vi "attribute_write_boolean.vi"(5 "Repeated Capability":string, 7 "Attribute":T1={"Identifier"="", "Descriptive name"="", "Data Type"=enum."Integer 32", "Command"="", "Access"=2, "Range Table"="", "Read Callback"="", "Write Callback"="", "Range Callback"="", "Check Callback"="", "Rngtable Callback"="", "Coerce Callback"="", "Supported Models"="", "Instrument Options"="", "Repeated Capabilities"="", "Check Status Callback"="", "Index"=0, "Flag: OPC Wait"=FALSE, "Flag: Dont check status"=FALSE, "Flag: Cache Only"=FALSE} {"Access" items=["Read Only", "Write Only", "Read/Write"]}, 8 "error in":errorcluster, 10 "boolean in":bool, 11 "VISA resource name":refnum<visa-resource-name>) -> (0 "error out":errorcluster, 3 "VISA resource name out":refnum<visa-resource-name>)   [LabVIEW 2014, in "rszvl_rsidr_core.lvlib"]
uses:
  rszvl_rsidr_core.lvlib
  type_Attribute.ctl
  type_Attribute_Data_Type.ctl
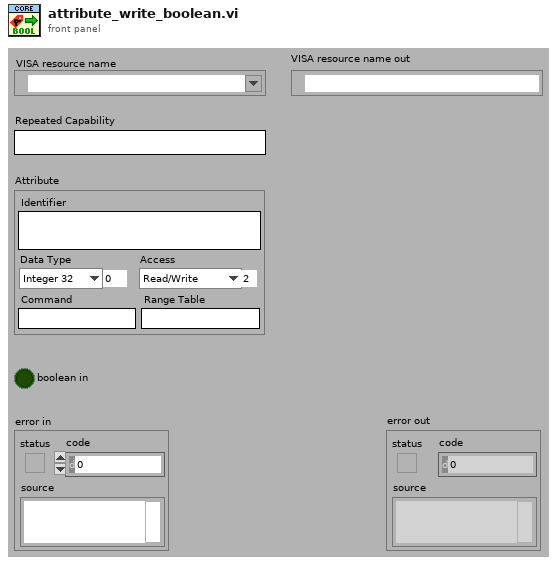
[diagram p1: front panel]
types:
  T1 = typedef "rszvl_rsidr_core.lvlib/type_Attribute.ctl" = cluster{"Identifier":string, "Descriptive name":string, "Data Type":T2, "Command":string, "Access":u16, "Range Table":string, "Read Callback":string, "Write Callback":string, "Range Callback":string, "Check Callback":string, "Rngtable Callback":string, "Coerce Callback":string, "Supported Models":string, "Instrument Options":string, "Repeated Capabilities":string, "Check Status Callback":string, "Index":i32, "Flag: OPC Wait":bool, "Flag: Dont check status":bool, "Flag: Cache Only":bool}
  T2 = typedef "rszvl_rsidr_core.lvlib/type_Attribute_Data_Type.ctl" = enum16{"Integer 32", "Double", "String", "Boolean", "None", "Integer 64"}
  T3 = typedef "rszvl_rsidr_core.lvlib/type_Session_Data.ctl" = cluster{"Instr type":string, "Instr type for err. msg.":string, "Installed Options":string[], "OPC Timeout":i32, "Query Instrument Status":bool, "Check Range":bool, "Check Options":bool, "Add LF to Write":bool, "Simulate":bool, "Logging":bool, "Logging params":variant, "Interface Type":enum16{"Unknown", "GPIB", "VXI", "GPIB_VXI", "ASRL", "PXI", "TCPIP", "USB", "SOCKET"}, "Fast Sweep":i32, "AdditionalFlags":i32, "WaitBeforeWrite":i32, "WaitBeforeRead":i32, "BinDataChunkSize":i64}
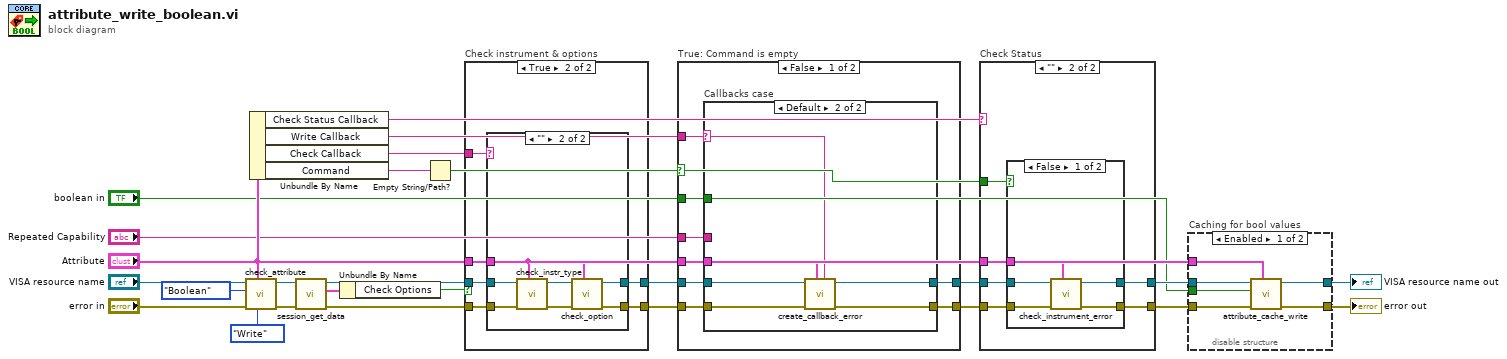
[diagram p0: block diagram]
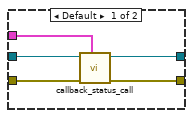
[diagram p2: hidden frame]
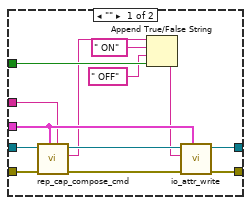
[diagram p4: hidden frame]
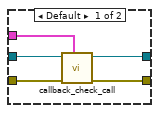
[diagram p7: hidden frame]
diagram:
  n1 = call "check_attribute.vi"("Access"=enum16{"Read", "Write"}."Write", "Attribute"="Attribute", "error in"="error in", "Data Type"=type_Attribute_Data_Type."Boolean", "VISA resource name"="VISA resource name") -> ("error out"=w13:errorcluster, "VISA resource name out"=w14:refnum<visa-resource-name>)  [unwired: 5 in]
  n2 = Unbundle By Name("Attribute") -> ("Check Status Callback"=w2:string, "Write Callback"=w15:string, "Check Callback"=w16:string, "Command"=w1:string)
  n3 = call "session_get_data.vi"("error in"=w13, "VISA resource name"=w14) -> ("error out"=w11:errorcluster, "Session User Data out"=w9:T3, "VISA resource name out"=w12:refnum<visa-resource-name>)  [unwired: 7 in]
  n4 = Unbundle By Name(w9) -> ("Check Options"=w10:bool)
  n5 = Empty String/Path?(string/path=w1) -> (empty?=w26:bool)
  n6 = case "Check instrument & options" shown="True" w10 {
    tunnel: [w28 w34] -> w7
    tunnel: [w27 w33] -> w6
    tunnel: "Attribute" -> [_ w32]
    tunnel: w16 -> [_ w31]
    tunnel: w12 -> [w28 w30]
    tunnel: w11 -> [w27 w29]
    frame False {
    }
    frame True {
      n7 = case shown="\"\"" w31 {
        tunnel: [w38 w44] -> w34
        tunnel: [w36 w43] -> w33
        tunnel: w29 -> [w37 w42]
        tunnel: w32 -> [w35 w40]
        tunnel: w30 -> [w39 w41]
        frame Default {
          n8 = call "callback_check_call.vi"("Attribute"=w35, "error in"=w37, "VISA resource name"=w39) -> ("error out"=w36:errorcluster, "VISA resource name out"=w38:refnum<visa-resource-name>)  [unwired: 7 in]
        }
        frame "" {
          n9 = call "check_instr_type.vi"("Attribute"=w40, "error in"=w42, "VISA resource name"=w41) -> ("error out"=w46:errorcluster, "VISA resource name out"=w45:refnum<visa-resource-name>)  [unwired: 6 in, 1 out]
          n10 = call "check_option.vi"("Attribute"=w40, "error in"=w46, "VISA resource name"=w45) -> ("error out"=w43:errorcluster, "VISA resource name out"=w44:refnum<visa-resource-name>)  [unwired: 7 in]
        }
      }
    }
  }
  n11 = case "True: Command is empty" shown="False" w26 {
    tunnel: "Repeated Capability" -> [w54 _]
    tunnel: w6 -> [w53 w74]
    tunnel: w7 -> [w52 w75]
    tunnel: "boolean in" -> [w51 _]
    tunnel: "Attribute" -> [w50 _]
    tunnel: [w49 w75] -> w3
    tunnel: [w48 w74] -> w4
    tunnel: w15 -> [w47 _]
    frame False {
      n12 = case "Callbacks case" shown="Default" w47 {
        selector: w47 -> [_ w68]
        tunnel: w51 -> [w61 _]
        tunnel: w52 -> [w66 w72]
        tunnel: w53 -> [w64 w73]
        tunnel: w54 -> [w59 _]
        tunnel: [w63 w70] -> w49
        tunnel: [w62 w71] -> w48
        tunnel: w50 -> [w60 w69]
        frame "" {
          n13 = call "rep_cap_compose_cmd.vi"("Repeated Capability"=w59, "Attribute"=w60, "error in"=w64, "VISA resource name"=w66) -> ("error out"=w65:errorcluster, "Command out"=w55:string, "VISA resource name out"=w67:refnum<visa-resource-name>)  [unwired: 5 in]
          n14 = Append True/False String(1:w61, 2:" OFF", 3:" ON", 4:w55) -> (0:w57:string)
          n15 = call "io_attr_write.vi"("Attribute"=w60, "error in"=w65, "write buffer"=w57, "VISA resource name"=w67) -> ("error out"=w62:errorcluster, "VISA resource name out"=w63:refnum<visa-resource-name>)  [unwired: 6 in]
        }
        frame Default {
          n16 = call "create_callback_error.vi"("Callback Name"=w68, "Attribute"=w69, "error in"=w73, "VISA resource name"=w72) -> ("error out"=w71:errorcluster, "VISA resource name out"=w70:refnum<visa-resource-name>)  [unwired: 6 in]
        }
      }
    }
    frame True {
    }
  }
  n17 = case "Check Status" shown="\"\"" w2 {
    tunnel: w4 -> [w80 w85]
    tunnel: [w79 w84] -> w25
    tunnel: [w78 w83] -> w24
    tunnel: w3 -> [w77 w86]
    tunnel: "Attribute" -> [w76 w82]
    tunnel: w26 -> [_ w81]
    frame Default {
      n18 = call "callback_status_call.vi"("Attribute"=w76, "error in"=w80, "VISA resource name"=w77) -> ("error out"=w79:errorcluster, "VISA resource name out"=w78:refnum<visa-resource-name>)  [unwired: 7 in]
    }
    frame "" {
      n19 = case shown="False" w81 {
        tunnel: w86 -> [w91 w93]
        tunnel: w85 -> [w90 w92]
        tunnel: [w89 w92] -> w84
        tunnel: [w88 w93] -> w83
        tunnel: w82 -> [w87 _]
        frame False {
          n20 = call "check_instrument_error.vi"("Attribute"=w87, "error in"=w90, "VISA resource name"=w91) -> ("error out"=w89:errorcluster, "VISA resource name out"=w88:refnum<visa-resource-name>)  [unwired: 7 in]
        }
        frame True {
        }
      }
    }
  }
  n21 = disable-structure "Caching for bool values" shown="Enabled" {
    disable-tunnel: [w99 w101] -> w19
    disable-tunnel: [w98 w100] -> w18
    disable-tunnel: w25 -> [w97 w100]
    disable-tunnel: w24 -> [w96 w101]
    disable-tunnel: "boolean in" -> [w95 _]
    disable-tunnel: "Attribute" -> [w94 _]
    frame Enabled {
      n22 = call "attribute_cache_write.vi"("Attribute"=w94, "error in"=w97, "Value in"=w95, "VISA resource name"=w96) -> ("error out"=w98:errorcluster, "VISA resource name out"=w99:refnum<visa-resource-name>)  [unwired: 6 in]
    }
    frame Disabled {
    }
  }
  "error out" <- w18
  "VISA resource name out" <- w19
